vi "ai and ao debug (rt).vi"() -> ()   [LabVIEW 2013]
uses:
  <vilib>/Platform/TimedLoop/XDataNode/timing_clust.ctl
  <vilib>/Platform/TimedLoop/XDataNode/nitl_modes.ctl
  <vilib>/Platform/TimedLoop/XDataNode/wakeup.ctl
  <vilib>/FPGAPlugInAG/sbRIO-9626/niLvFpga_Open_sbRIO-9626.vi
  <vilib>/rvi/interface/common/dynamic/niFpgaDynamicAddResources.vi
  <vilib>/FPGAPlugInAG/Dynamic/niLvFpga_Run_Dynamic.vi
  <vilib>/rvi/interface/common/niFpgaWaitOnOcc.vi
  <vilib>/Utility/error.llb/Error Cluster From Error Code.vi
  <vilib>/rvi/errors/niLvFpgaAdjustHostInterfaceError.vi
  <vilib>/FPGAPlugInAG/Dynamic/niLvFpga_Close_Dynamic.vi
  <vilib>/Platform/TimedLoop/XDataNode/XDataNode.xnode
  <vilib>/rvi/interface/nirviOpenFPGA/nirviOpenFPGA.xnode
  FPGA Bitfiles/TIsbRIO_FPGATarget_aiandaodebug(fpg_wLTa3gHS5zI.lvbitx
  FPGA/ai and ao debug (fpga).vi
  <vilib>/rvi/interface/nirviMethod/nirviMethod.xnode
  <vilib>/rvi/interface/nirviReadWriteControl/nirviReadWriteControl.xnode
  <vilib>/rvi/interface/nirviCloseFPGA/nirviCloseFPGA.xnode
  <vilib>/rvi/interface/Simulation/niFpgaSimulationCallBeginRW.vi
  <vilib>/Platform/TimedLoop/XDataNode/XDNodeRunTimeDep.lvlib
  NiFpgaLv.dll
  <vilib>/ptbypt/NI_PtbyPt.lvlib
panel:
  out "mean":dbl format="%0.2f"
  out "Analog Inputs":sgl[](array[numeric])
  out "CFR":u64 format="%.0x"
  out "Analog Inputs (raw)":u16[](array[numeric])
  in  "stop 2":bool
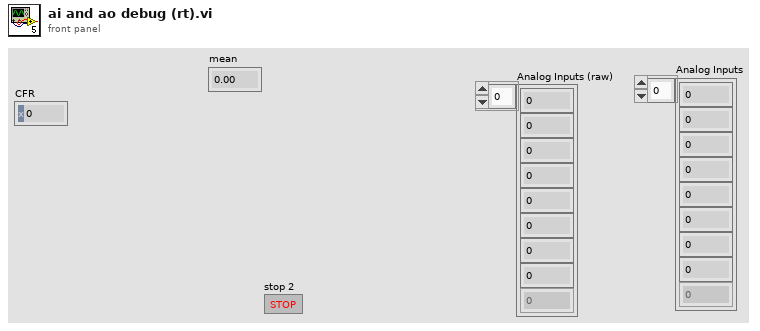
[diagram p1: front panel]
types:
  T1 = cluster{"Divide Value":u8, "Transfer Length (bits)":u8, "CS Asserted Polarity":bool, "Clock Polarity (CPOL)":bool, "Clock Phase (CPHA)":bool, "Lengthen MISO Setup":bool, "Direction Change Bit":u8, "MOSI Starts as Output":bool, "Tristatable MOSI":bool}
  T2 = typedef "XDNodeRunTimeDep.lvlib/timing_clust.ctl" = cluster{"Expected End [f-1]":u64, "Actual End [f-1]":u64, "Finished Late? [f-1]":bool, "Expected End [i-1]":u64, "Actual End [i-1]":u64, "Finished Late? [i-1]":bool, "Expected Start [i]":u64, "Actual Start [i]":u64, "Expected Start [f]":u64, "Actual Start [f]":u64, "Source Name":string, "Structure Name":string, "Period":i64, "Deadline":i64, "Offset":i64, "Start":i64, "Priority":i32, "Timeout":i32, "Mode":T3, "Wakeup Reason":T4, "Error":errorcluster, "Source Type":string, "Secondary Source Type":string, "Global End Time":u64, "Global Start Time":u64, "Frame Duration":u64, "Iteration Duration":u64, "Assigned CPU":i32, "I/O Scan Engine Mode":u32}
  T3 = typedef "XDNodeRunTimeDep.lvlib/nitl_modes.ctl" = enum32{"No Change", "Process missed periods, maintain original phase", "Discard missed periods, maintain original phase", "Process missed periods, ignore original phase", "Discard missed periods, ignore original phase"}
  T4 = typedef "XDNodeRunTimeDep.lvlib/wakeup.ctl" = enum32{"Normal", "Aborted", "Asynchronous wakeup", "Timing source error", "Timed loop error", "Timeout"}
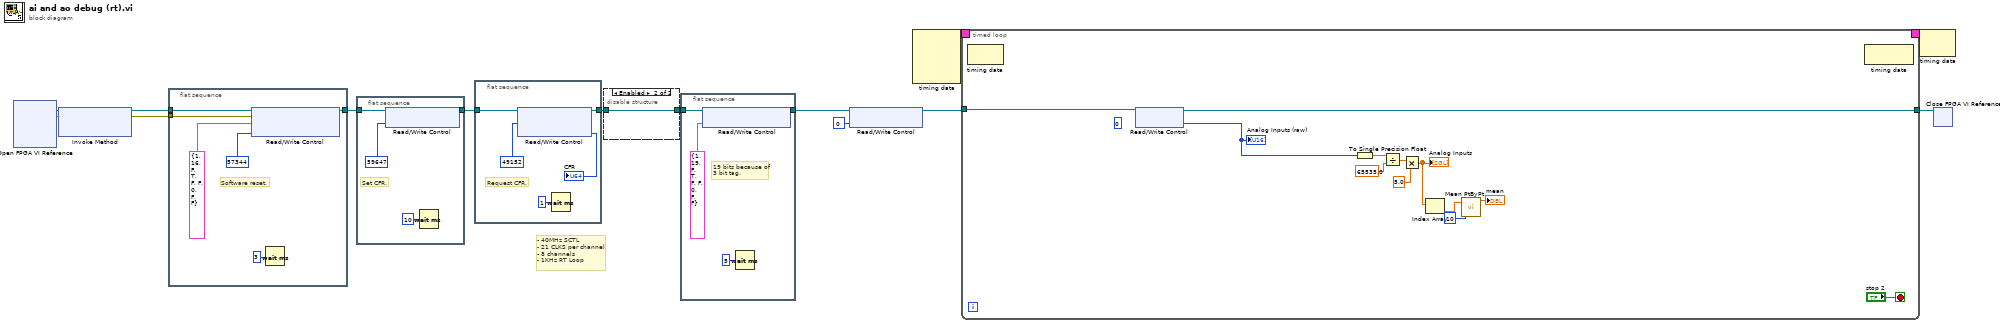
[diagram p0: block diagram]
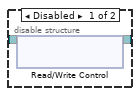
[diagram p2: hidden frame]
diagram:
  # "- 40MHz SCTL\n- 21 CLKS per channel\n- 8 channels\n- 1KHz RT Loop"
  n1 = xnode "Open FPGA VI Reference"() -> ("FPGA VI Reference Out"=w9:refnum<k20>, "error out"=w8:errorcluster)  [unwired: 2 in]
  n2 = xnode "Invoke Method"("FPGA VI Reference In"=w9, "error in"=w8) -> ("FPGA VI Reference Out"=w11:refnum<k20>, "error out"=w10:errorcluster)  [unwired: 1 in]
  n3 = flat-sequence {
    tunnel: w11 -> [w20]
    tunnel: w10 -> [w19]
    tunnel: [w16] -> w4
    frame #0 {
      # "Software reset."
      n4 = xnode "Read/Write Control"("FPGA VI Reference In"=w20, "error in"=w19, "Onboard AI SPI Settings"=T1 {"Divide Value"=1, "Transfer Length (bits)"=16, "CS Asserted Polarity"=FALSE, "Clock Polarity (CPOL)"=TRUE, "Clock Phase (CPHA)"=FALSE, "Lengthen MISO Setup"=FALSE, "Direction Change Bit"=0, "MOSI Starts as Output"=FALSE, "Tristatable MOSI"=FALSE} ("Master Settings"), "Onboard AI Data In"=u64 57344 ("data to write")) -> ("FPGA VI Reference Out"=w16:refnum<k20>)  [unwired: 1 out]
      n5 = Wait (ms)(milliseconds to wait=u32 3) -> ()  [unwired: 1 out]
    }
  }
  n6 = flat-sequence {
    tunnel: [w24] -> w6
    tunnel: w4 -> [w22]
    frame #0 {
      # "Set CFR."
      n7 = xnode "Read/Write Control"("FPGA VI Reference In"=w22, "Onboard AI Data In"=u64 59647 ("data to write")) -> ("FPGA VI Reference Out"=w24:refnum<k20>)  [unwired: 1 in, 1 out]
      n8 = Wait (ms)(milliseconds to wait=u32 10) -> ()  [unwired: 1 out]
    }
  }
  n9 = flat-sequence {
    tunnel: [w29] -> w7
    tunnel: w6 -> [w27]
    frame #0 {
      # "Request CFR."
      n10 = xnode "Read/Write Control"("FPGA VI Reference In"=w27, "Onboard AI Data In"=u64 49152 ("data to write")) -> ("FPGA VI Reference Out"=w29:refnum<k20>, "Onboard AI Data"=→"CFR":u64)  [unwired: 1 in, 1 out]
      n11 = Wait (ms)(milliseconds to wait=u32 1) -> ()  [unwired: 1 out]
    }
  }
  n12 = disable-structure shown="Enabled" {
    disable-tunnel: w7 -> [w31 w32]
    disable-tunnel: [w30 w32] -> w5
    frame Disabled {
      n13 = xnode "Read/Write Control"("FPGA VI Reference In"=w31) -> ("FPGA VI Reference Out"=w30:refnum<k20>)  [unwired: 1 in, 2 out]
    }
    frame Enabled {
    }
  }
  n14 = flat-sequence {
    tunnel: [w35] -> w3
    tunnel: w5 -> [w34]
    frame #0 {
      # "19 bits because of\n3 bit tag."
      n15 = xnode "Read/Write Control"("FPGA VI Reference In"=w34, "Onboard AI SPI Settings"=T1 {"Divide Value"=1, "Transfer Length (bits)"=19, "CS Asserted Polarity"=FALSE, "Clock Polarity (CPOL)"=TRUE, "Clock Phase (CPHA)"=FALSE, "Lengthen MISO Setup"=FALSE, "Direction Change Bit"=0, "MOSI Starts as Output"=FALSE, "Tristatable MOSI"=FALSE} ("Master Settings")) -> ("FPGA VI Reference Out"=w35:refnum<k20>)  [unwired: 1 in, 1 out]
      n16 = Wait (ms)(milliseconds to wait=u32 5) -> ()  [unwired: 1 out]
    }
  }
  n17 = xnode "Read/Write Control"("FPGA VI Reference In"=w3, "Onboard AI Data In"=u64 0) -> ("FPGA VI Reference Out"=w2:refnum<k20>)  [unwired: 1 in, 1 out]
  n18 = node-c288() -> (w13:T2)  [unwired: 4 in]
  n19 = timed-loop {
    timing: w13 -> [_]
    timing-out: [_] -> w12
    tunnel: [w47] -> w14
    tunnel: w2 -> [w46]
    stop <- "stop 2" stop-if-true
    (unwired) u64 0 ("data to write")
    n20 = node-c288() -> ()  [unwired: 1 in, 1 out]
    n21 = xnode "Read/Write Control"("FPGA VI Reference In"=w46) -> ("FPGA VI Reference Out"=w47:refnum<k20>, "Onboard AI"=w41:u16[])  [unwired: 1 in, 1 out]
    "Analog Inputs (raw)" <- w41
    n22 = To Single Precision Float(number=w41) -> (single precision float=w42:sgl[])
    n23 = Divide(x=w42, y=sgl 65535.0 ("millisecond multiple")) -> (x/y=w44:sgl[])
    n24 = Multiply(x=w44, y=sgl 5.0 ("millisecond multiple")) -> (x*y=w40:sgl[])
    "Analog Inputs" <- w40
    n25 = Index Array(array=w40) -> (element=w39:sgl)  [unwired: 1 in]
    n26 = call <vilib>:"Mean PtByPt.vi"("x"=w39, "sample length"=10) -> ("mean"=→"mean":dbl)  [unwired: 2 in, 1 out]
    n27 = node-c288() -> ()  [unwired: 1 in, 1 out]
  }
  n28 = node-c288(w12) -> ()  [unwired: 1 out]
  n29 = xnode "Close FPGA VI Reference"("FPGA VI Reference In"=w14) -> ()  [unwired: 1 in, 1 out]
